vi "GetDeviceAddress.vi"(8 "error in (no error)":errorcluster, 10 "DeviceKey In":string, 11 "CmdLib In":refnum<k24>) -> (0 "error out":errorcluster, 1 "Device Address":i32, 2 "DeviceKey Out":string, 3 "CmdLib Out":refnum<k24>)   [LabVIEW 2024]
uses:
  C:/Development/rimas/RIMAS/Focus/PicoMotor/CmdLib.dll
  CmdLib.dll
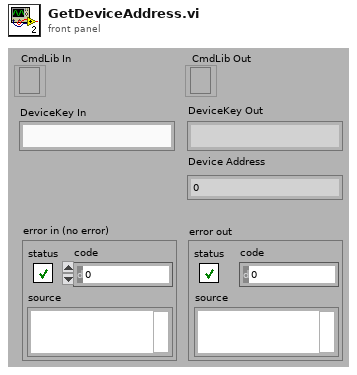
[diagram p1: front panel]
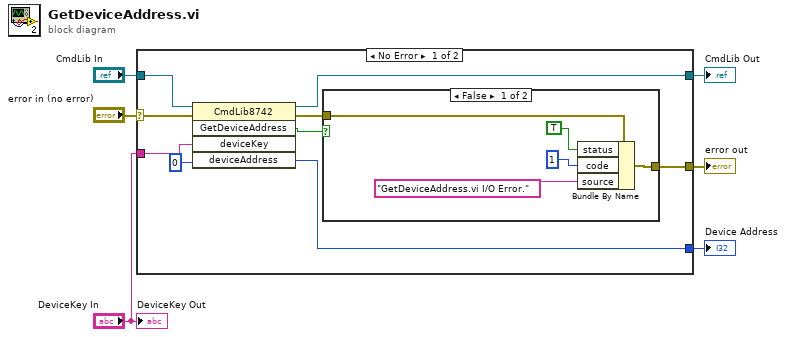
[diagram p0: block diagram]
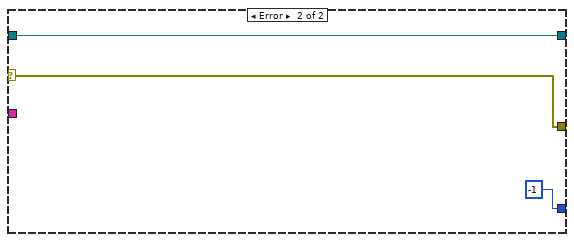
[diagram p3: hidden frame]
diagram:
  n1 = case shown="No Error" "error in (no error)" {
    selector: "error in (no error)" -> [w12 w23]
    tunnel: "CmdLib In" -> [w15 w24]
    tunnel: [w14 w24] -> w5
    tunnel: "DeviceKey In" -> [w13 _]
    tunnel: [w9 w23] -> w2
    tunnel: [w8 -1] -> w1
    frame No Error {
      n2 = invoke class="CmdLib8742" method="GetDeviceAddress"(reference=w15, error in=w12, "deviceKey"=w13, "deviceAddress"=0) -> (reference out=w14:refnum<k24>, error out=w10:errorcluster, "GetDeviceAddress"=w11:bool, "deviceAddress"=w8:i32)  [unwired: 1 in, 1 out]
      n3 = case shown="False" w11 {
        tunnel: w10 -> [w20 w21]
        tunnel: [w19 w21] -> w9
        frame False {
          n4 = Bundle By Name(cluster=w20, "status"=TRUE, "code"=1, "source"="GetDeviceAddress.vi I/O Error.") -> (w19:errorcluster)
        }
        frame True {
        }
      }
    }
    frame Error {
    }
  }
  "error out" <- w2
  "CmdLib Out" <- w5
  "Device Address" <- w1
  "DeviceKey Out" <- "DeviceKey In"
